vi "RX.vi"(2 "v Ctrl in":refnum<class "CtrlLine.lvclass">, 7 "QuWire in":refnum<class "QuWire.lvclass">, 11 "theta":dbl, 13 "^ Ctrl in":refnum<class "CtrlLine.lvclass">) -> (8 "QuWire out":refnum<class "QuWire.lvclass">)   [LabVIEW 2020]
doc: "Rx Gate\n\nRotates the target qubit by an arbitrary angle theta (radians) around the x-axis."
uses:
  QuSim/QuWire/QuWire.lvclass
  QuSim/QuWire/CtrlLine/CtrlLine.lvclass
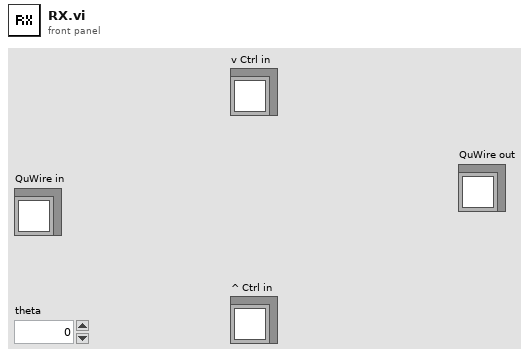
[diagram p1: front panel]
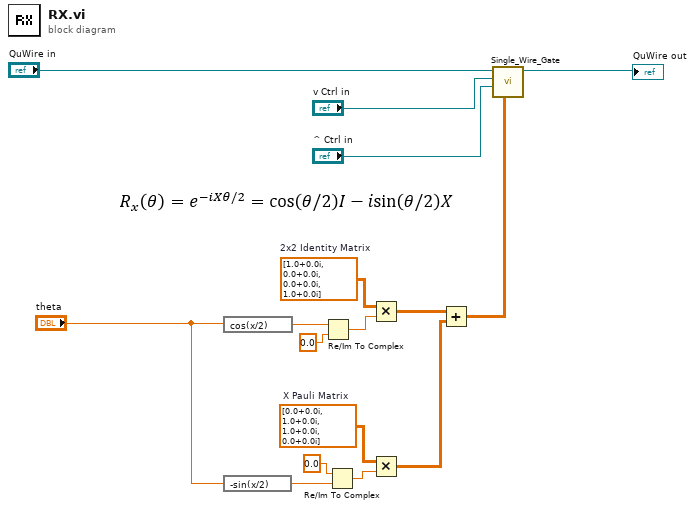
[diagram p0: block diagram]
diagram:
  w8 = cdb[][] [[0.0+0.0i, 1.0+0.0i], [1.0+0.0i, 0.0+0.0i]]  # X Pauli Matrix
  w12 = cdb[][] [[1.0+0.0i, 0.0+0.0i], [0.0+0.0i, 1.0+0.0i]]  # 2x2 Identity Matrix
  n1 = expression code="cos(x/2)"("theta") -> (w11:dbl)
  n2 = expression code="-sin(x/2)"("theta") -> (w6:dbl)
  n3 = Re/Im To Complex(1:0.0 ("y"), 2:w11) -> (0:w4:cdb)
  n4 = Re/Im To Complex(1:w6, 2:0.0 ("x")) -> (0:w7:cdb)
  n5 = Multiply(x=w12, y=w4) -> (x*y=w3:cdb[][])
  n6 = Multiply(x=w8, y=w7) -> (x*y=w5:cdb[][])
  n7 = Add(x=w3, y=w5) -> (x+y=w2:cdb[][])
  n8 = call "Single_Wire_Gate.vi"("2x2 Unitary Matrix"=w2, "d CtrlLine in"="^ Ctrl in", "u CtrlLine in"="v Ctrl in", "QuWire in"="QuWire in") -> ("QuWire out"=→"QuWire out":refnum<class "QuWire.lvclass">)  [unwired: 6 in, 1 out]
